vi "Write File.vi"(8 "error in (no error)":errorcluster, 9 "Data":variant, 10 "datalog path (use dialog)":path, 11 "Switch File Interface in":refnum<class "Switch File Interface.lvclass">) -> (0 "error out":errorcluster)   [LabVIEW 2018, in "Switch System Explorer.lvlib" / "Switch File Interface.lvclass"]
uses:
  Switch Configuration.llb/Switch File Interface.lvclass
  Switch Configuration.llb/Switch CD Configuration.lvclass
  Switch Configuration.llb/PXI Card Config.lvclass
  C:/Users/jennifer.platt/Documents/Switch-Custom-Device - Copy/Built/Switch/Windows/Switch Configuration.llb/Switch Card Config.lvclass
  Switch Configuration.llb/SLSC Card Config.lvclass
  Switch Configuration.llb/Constants.vi
  Switch Configuration.llb/Switch Shared.lvlib
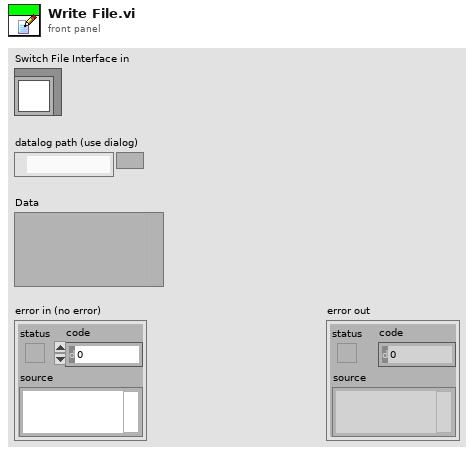
[diagram p1: front panel]
types:
  T1 = cluster{"Startup and Shutdown Options":cluster{"Set all values to default on startup":bool, "Stop execution on error":bool, "Set all values to default on exit":bool}, "Value out of range handling:":enum32{"default state", "maintain state", "Shutdown"}}
  T2 = cluster{"Version":string, "Tree":cluster{"Item Info":cluster{"Name":string, "Description":string, "GUID":string, "Is Channel":bool, "Channel":cluster{"Type":enum16{"Input", "Output"}, "Units":string, "Default Value":dbl, "Faultable":bool, "Scalable":bool}, "Is Waveform":bool, "Waveform":cluster{"Data Type":enum16{"Double", "Complex Double"}, "Units":string}}, "Parent Path":string[], "Properties":cluster{"Name":string, "Type":i32, "Value":variant}[]}[]}
  T3 = cluster{"Item Info":cluster{"Name":string, "Description":string, "GUID":string, "Is Channel":bool, "Channel":cluster{"Type":enum16{"Input", "Output"}, "Units":string, "Default Value":dbl, "Faultable":bool, "Scalable":bool}, "Is Waveform":bool, "Waveform":cluster{"Data Type":enum16{"Double", "Complex Double"}, "Units":string}}, "Parent Path":string[], "Properties":cluster{"Name":string, "Type":i32, "Value":variant}[]}[]
  T4 = cluster{"Name":string, "Type":i32, "Value":variant}[]
  T5 = cluster{"Name":string, "Type":i32, "Value":variant}
  T6 = cluster{"Set all values to default on startup":bool, "Stop execution on error":bool, "Set all values to default on exit":bool}
  T7 = enum32{"default state", "maintain state", "Shutdown"}
  T8 = cluster{"Device/Resource Name":string, "Alias":string, "Topology Name":string, "Driver Type":enum16{"PXI", "SLSC"}, "Route(F)/Relay(T)":bool, "Channel List":string[], "Relay List":string[], "Simulate?":bool, "SLSC Driver Settings":cluster{"Local(F)/Remote(T)":bool, "Host IP":string, "Port":i32}, "Continuous Reservation?":bool}
  T9 = cluster{"Local(F)/Remote(T)":bool, "Host IP":string, "Port":i32}
  T10 = cluster{"Channel Name":string, "State Configs":cluster{"State Value":dbl, "State Name":string, "Command Configs":cluster{"Card Alias":string, "Ch0/Relay":string, "Ch1":string, "Disconnect(F)/Connect(T)":bool}[]}[]}
  T11 = cluster{"State Value":dbl, "State Name":string, "Command Configs":cluster{"Card Alias":string, "Ch0/Relay":string, "Ch1":string, "Disconnect(F)/Connect(T)":bool}[]}[]
  T12 = cluster{"Card Alias":string, "Ch0/Relay":string, "Ch1":string, "Disconnect(F)/Connect(T)":bool}[]
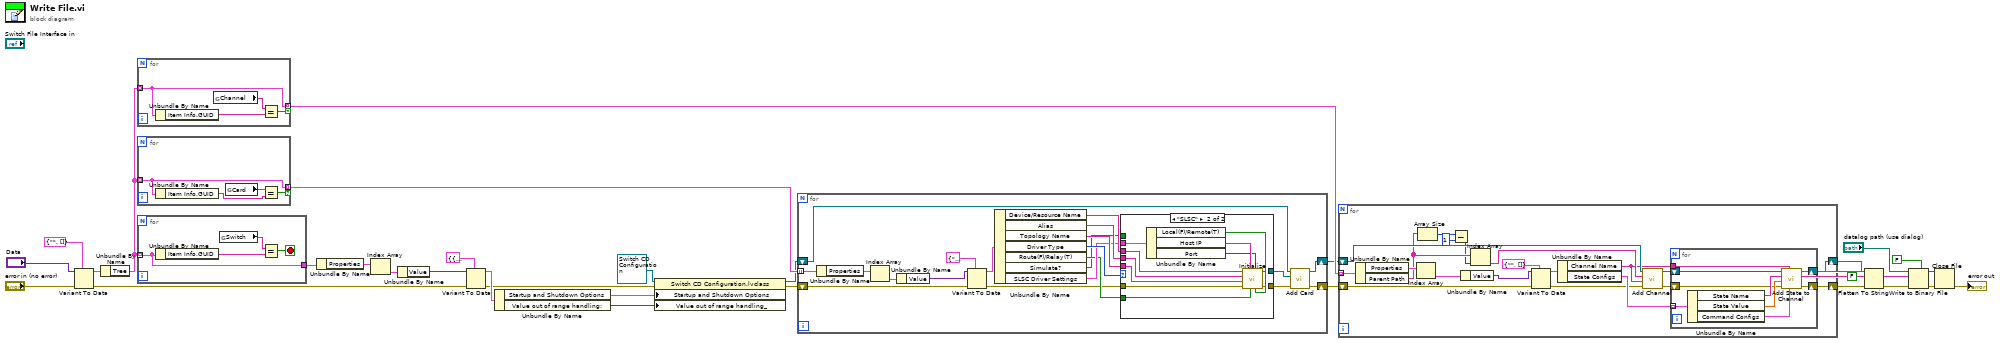
[diagram p0: block diagram]
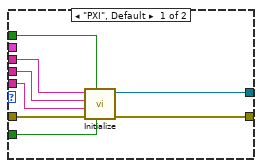
[diagram p2: hidden frame]
diagram:
  n1 = Variant To Data(error in="error in (no error)", type=T2 {"Version"="", "Tree"=[]} ("SysDef"), Variant="Data") -> (data=w30:T2, error out=w6:errorcluster)
  n2 = Unbundle By Name(w30) -> ("Tree"=w7:T3)
  n3 = for {
    tunnel: w7 -> [w34] mode=indexing
    tunnel: [w34] -> w19 mode=indexing if=w33
    n4 = Unbundle By Name(w34) -> ("Item Info.GUID"=w36:string)
    n5 = global read "Constants.vi" "Channel"() -> (w35:string)
    n6 = Equal?(x=w35, y=w36) -> (x = y?=w33:bool)
  }
  n7 = for {
    tunnel: w7 -> [w38] mode=indexing
    tunnel: [w38] -> w20 mode=indexing if=w37
    n8 = Unbundle By Name(w38) -> ("Item Info.GUID"=w40:string)
    n9 = global read "Constants.vi" "Card"() -> (w39:string)
    n10 = Equal?(x=w39, y=w40) -> (x = y?=w37:bool)
  }
  n11 = for {
    tunnel: w7 -> [w41] mode=indexing
    tunnel: [w41] -> w29
    stop <- w42 stop-if-true
    n12 = Unbundle By Name(w41) -> ("Item Info.GUID"=w44:string)
    n13 = global read "Constants.vi" "Switch"() -> (w43:string)
    n14 = Equal?(x=w43, y=w44) -> (x = y?=w42:bool)
  }
  n15 = Unbundle By Name(w29) -> ("Properties"=w28:T4)
  n16 = Index Array(array=w28) -> (element=w27:T5)  [unwired: 1 in]
  n17 = Unbundle By Name(w27) -> ("Value"=w25:variant)
  n18 = Variant To Data(error in=w6, type=T1 {"Startup and Shutdown Options"={"Set all values to default on startup"=FALSE, "Stop execution on error"=FALSE, "Set all values to default on exit"=FALSE}, "Value out of range handling:"=enum."default state"} ("Switch Device Data"), Variant=w25) -> (data=w24:T1, error out=w5:errorcluster)
  n19 = Unbundle By Name(w24) -> ("Startup and Shutdown Options"=w22:T6, "Value out of range handling:"=w21:T7)
  n20 = property class="Switch CD Configuration.lvclass"(reference=refnum<class "Switch CD Configuration.lvclass"> refnum ("Switch CD Configuration.lvclass"), error in=w5, "Startup and Shutdown Options"=w22, "Value out of range handling_"=w21) -> (reference out=w18:refnum<class "Switch CD Configuration.lvclass">, error out=w4:errorcluster)
  n21 = for {
    tunnel: w20 -> [w61] mode=indexing
    shift-right: [w49] -> w17
    shift-left: w18 -> [w50]
    shift-right: [w45] -> w3
    shift-left: w4 -> [w48]
    n22 = Unbundle By Name(w61) -> ("Properties"=w62:T4)
    n23 = Index Array(array=w62) -> (element=w63:T5)  [unwired: 1 in]
    n24 = Unbundle By Name(w63) -> ("Value"=w64:variant)
    n25 = Variant To Data(error in=w48, type=T8 {"Device/Resource Name"="", "Alias"="", "Topology Name"="", "Driver Type"=enum."PXI", "Route(F)/Relay(T)"=FALSE, "Channel List"=[], "Relay List"=[], "Simulate?"=FALSE, "SLSC Driver Settings"={"Local(F)/Remote(T)"=FALSE, "Host IP"="", "Port"=0}, "Continuous Reservation?"=FALSE} ("Device Information"), Variant=w64) -> (data=w59:T8, error out=w47:errorcluster)
    n26 = Unbundle By Name(w59) -> ("Device/Resource Name"=w57:string, "Alias"=w56:string, "Topology Name"=w55:string, "Driver Type"=w58:enum16{"PXI", "SLSC"}, "Route(F)/Relay(T)"=w53:bool, "Simulate?"=w52:bool, "SLSC Driver Settings"=w54:T9)
    n27 = case shown="\"SLSC\"" w58 {
      tunnel: w57 -> [w72 w83]
      tunnel: w56 -> [w71 w82]
      tunnel: w55 -> [w70 w81]
      tunnel: w54 -> [_ w80]
      tunnel: w53 -> [w68 w76]
      tunnel: w52 -> [w69 _]
      tunnel: [w67 w75] -> w51
      tunnel: w47 -> [w66 w74]
      tunnel: [w65 w73] -> w46
      frame "PXI", Default {
        n28 = call "Initialize.vi"("Route(F)/Relay(T)"=w68, "Simulate?"=w69, "error in (no error)"=w66, "Topology"=w70, "Alias"=w71, "Device/Resource Name"=w72) -> ("error out"=w65:errorcluster, "PXI Card Config"=w67:refnum<class "PXI Card Config.lvclass">)  [unwired: 4 in]
      }
      frame "SLSC" {
        n29 = Unbundle By Name(w80) -> ("Local(F)/Remote(T)"=w79:bool, "Host IP"=w78:string, "Port"=w77:i32)
        n30 = call "Initialize.vi"("Local(F)_Remote(T)"=w79, "Port"=w77, "Route(F)/Relay(T)"=w76, "Host IP"=w78, "error in (no error)"=w74, "Topology"=w81, "Alias"=w82, "Device/Resource Name"=w83) -> ("error out"=w73:errorcluster, "SLSC Card Config out"=w75:refnum<class "SLSC Card Config.lvclass">)  [unwired: 2 in]
      }
    }
    n31 = call "Add Card.vi"("error in (no error)"=w46, "Switch Card Config"=w51, "Switch CD Configuration"=w50) -> ("error out"=w45:errorcluster, "Switch CD Configuration"=w49:refnum<class "Switch CD Configuration.lvclass">)  [unwired: 7 in]
  }
  n32 = for {
    tunnel: w19 -> [w100] mode=indexing
    shift-right: [w92] -> w10
    shift-left: w17 -> [w97]
    shift-right: [w88] -> w2
    shift-left: w3 -> [w91]
    n33 = Unbundle By Name(w100) -> ("Properties"=w101:T4, "Parent Path"=w87:string[])
    n34 = Index Array(array=w101) -> (element=w102:T5)  [unwired: 1 in]
    n35 = Array Size(array=w87) -> (size(s)=w86:i32)
    n36 = Subtract(x=w86, y=1) -> (x-y=w84:i32)
    n37 = Unbundle By Name(w102) -> ("Value"=w103:variant)
    n38 = Index Array(array=w87, index=w84) -> (element=w96:string)
    n39 = Variant To Data(error in=w91, type=T10 {"Channel Name"="", "State Configs"=[]} ("Channel Config"), Variant=w103) -> (data=w99:T10, error out=w90:errorcluster)
    n40 = Unbundle By Name(w99) -> ("Channel Name"=w93:string, "State Configs"=w94:T11)
    n41 = call "Add Channel.vi"("error in (no error)"=w90, "Name"=w93, "Group Name"=w96, "Switch CD Configuration"=w97) -> ("error out"=w89:errorcluster, "Switch CD Configuration"=w95:refnum<class "Switch CD Configuration.lvclass">)  [unwired: 5 in, 1 out]
    n42 = for {
      tunnel: w94 -> [w111] mode=indexing
      tunnel: w93 -> [w107]
      shift-right: [w106] -> w92
      shift-left: w95 -> [w112]
      shift-right: [w104] -> w88
      shift-left: w89 -> [w105]
      n43 = Unbundle By Name(w111) -> ("State Name"=w110:string, "State Value"=w109:dbl, "Command Configs"=w108:T12)
      n44 = call "Add State to Channel.vi"("Command Configs"=w108, "Channel Name"=w107, "error in (no error)"=w105, "Value"=w109, "State Name"=w110, "Switch CD Configuration"=w112) -> ("error out"=w104:errorcluster, "Switch CD Configuration"=w106:refnum<class "Switch CD Configuration.lvclass">)  [unwired: 4 in]
    }
  }
  n45 = Flatten To String(anything=w10, prepend array or string size? (T)=FALSE, error in (no error)=w2) -> (data string=w13:string, error out=w14:errorcluster)  [unwired: 1 in, 1 out]
  n46 = Write to Binary File(file (use dialog)="datalog path (use dialog)", data=w13, error in=w14, 5:FALSE ("prepend array or string size? (T)")) -> (refnum out=w15:refnum<file>, error out=w16:errorcluster)  [unwired: 2 in, 1 out]
  n47 = Close File(refnum=w15, error in=w16) -> (error out=→"error out":errorcluster)  [unwired: 1 out]
